vi "kvaly.vi"   [LabVIEW 2017]
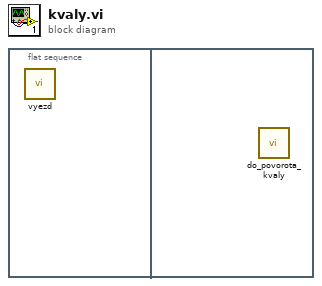
[diagram p0: block diagram]
diagram:
  n1 = flat-sequence {
    frame #0 {
      n2 = call "vyezd.vi"() -> ()  [unwired: 12 in]
    }
    frame #1 {
      n3 = call "do_povorota_kvaly.vi"() -> ()  [unwired: 12 in]
    }
  }
